vi "Configure Instrument Locations.vi"(5 "V-Meter":refnum<visa-resource-name>, 7 "Switch":refnum<visa-resource-name>, 8 "error in (no error)":errorcluster, 9 "Magnet":refnum<visa-resource-name>, 10 "I-SRC":refnum<visa-resource-name>, 11 "Ammeter":refnum<visa-resource-name>) -> (0 "error out":errorcluster)   [LabVIEW 2016, in "Hall Effect Library.lvlib"]
uses:
  Hall Effect Library.lvlib
  Private/Global Variables/Instrument Locations.vi
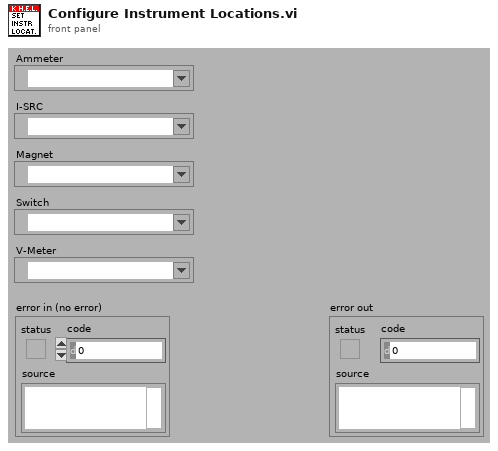
[diagram p1: front panel]
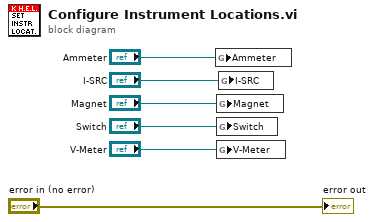
[diagram p0: block diagram]
diagram:
  n1 = global write "Instrument Locations.vi" "Ammeter"("Ammeter") -> ()
  n2 = global write "Instrument Locations.vi" "Magnet"("Magnet") -> ()
  n3 = global write "Instrument Locations.vi" "Switch"("Switch") -> ()
  n4 = global write "Instrument Locations.vi" "V-Meter"("V-Meter") -> ()
  n5 = global write "Instrument Locations.vi" "I-SRC"("I-SRC") -> ()
  "error out" <- "error in (no error)"
